vi "SendCommand.vi"(8 "error in (no error)":errorcluster, 10 "String to Send":string, 11 "OXY_SCPI Reseource In":refnum<visa-resource-name>) -> (0 "error out":errorcluster, 3 "OXY_SCPI Reseource Out":refnum<visa-resource-name>)   [LabVIEW 2018, in "OXYGEN.lvlib"]
uses:
  OXYGEN.lvlib
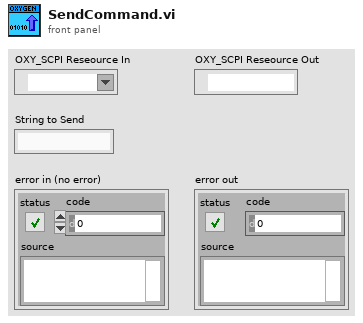
[diagram p1: front panel]
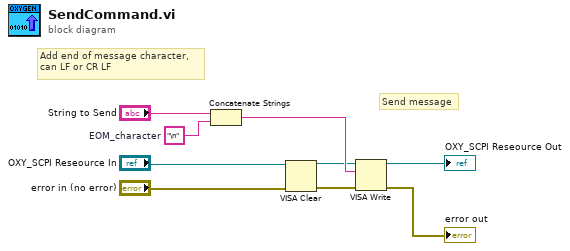
[diagram p0: block diagram]
diagram:
  w5 = "\n"  # EOM_character
  # "Send message"
  # "Add end of message character,\ncan LF or CR LF"
  n1 = Concatenate Strings("String to Send", w5) -> (w6:string)
  n2 = VISA Clear(VISA resource name="OXY_SCPI Reseource In", error in (no error)="error in (no error)") -> (VISA resource name out=w3:refnum<visa-resource-name>, error out=w4:errorcluster)
  n3 = VISA Write(VISA resource name=w3, write buffer=w6, error in (no error)=w4) -> (VISA resource name out=→"OXY_SCPI Reseource Out":refnum<visa-resource-name>, error out=→"error out":errorcluster)  [unwired: 1 out]
